vi "Init.vi"(8 "error in (no error)":errorcluster, 10 "Node Info":T1, 11 "Name":string) -> (0 "error out":errorcluster, 3 "Node out":refnum<class "Node.lvclass">)   [LabVIEW 2020, in "Vecto.lvlib" / "Node.lvclass"]
uses:
  Node.lvclass
  Node Info.ctl
  Node.lvclass/Node.ctl
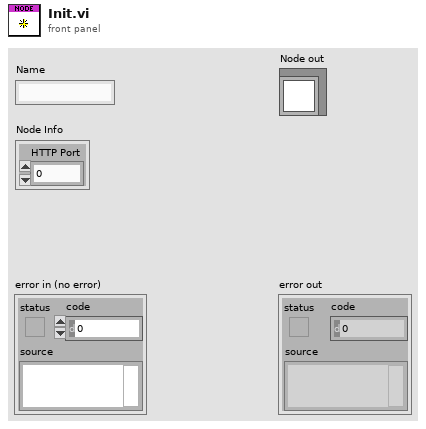
[diagram p1: front panel]
types:
  T1 = typedef "Vecto.lvlib/Node.lvclass/Node Info.ctl" = cluster{"HTTP Port":u16}
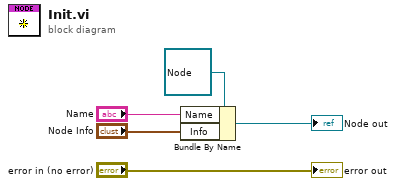
[diagram p0: block diagram]
diagram:
  n1 = Bundle By Name(cluster=refnum<class "Node.lvclass"> refnum ("Node in"), "Name"="Name", "Info"="Node Info") -> (→"Node out":refnum<class "Node.lvclass">)
  "error out" <- "error in (no error)"
